vi "Mask for png matrix.vi"(11 "24-bit pixmap in":u32[][](array[numeric])) -> (3 "24-bit pixmap out":u32[][](array[numeric]))   [LabVIEW 2017]
panel:
  in  "ColorMask":u32(colorbox)
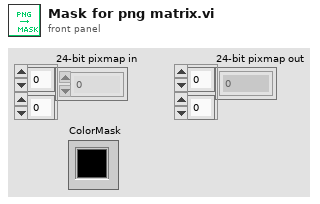
[diagram p1: front panel]
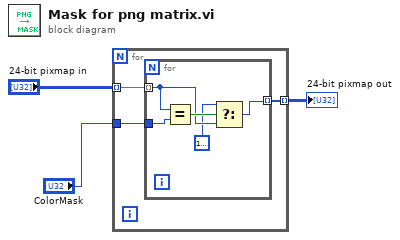
[diagram p0: block diagram]
diagram:
  n1 = for {
    tunnel: "24-bit pixmap in" -> [w6] mode=indexing
    tunnel: "ColorMask" -> [w5]
    tunnel: [w4] -> w1 mode=indexing
    n2 = for {
      tunnel: w6 -> [w8] mode=indexing
      tunnel: w5 -> [w11]
      tunnel: [w9] -> w4 mode=indexing
      n3 = Equal?(x=w8, y=w11) -> (x = y?=w10:bool)
      n4 = Select(t=u32 16777216 ("ColorMask"), s=w10, f=w8) -> (s? t:f=w9:u32)
    }
  }
  "24-bit pixmap out" <- w1
